vi "factorial function-for-while.vi"() -> ()   [LabVIEW 2023]
panel:
  out "String 2":string
  out "String":string
  out "String":string
  out "Numeric 6":i32
  in  "Numeric 5":i32
  in  "Numeric 3":i32
  out "Numeric 4":i32
  out "Numeric 2":i32
  in  "Numeric":i32
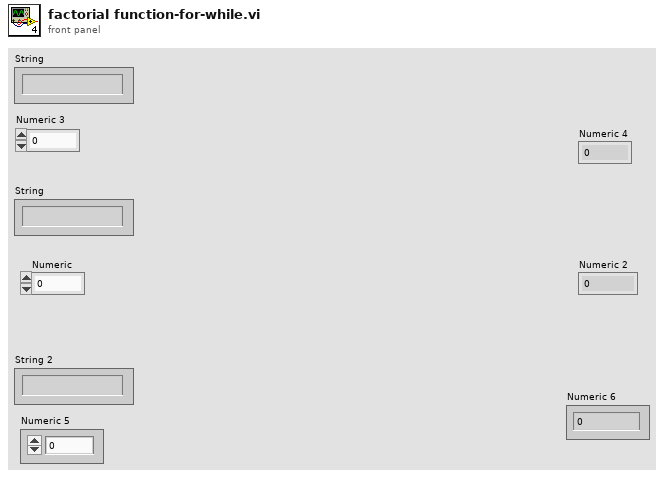
[diagram p1: front panel]
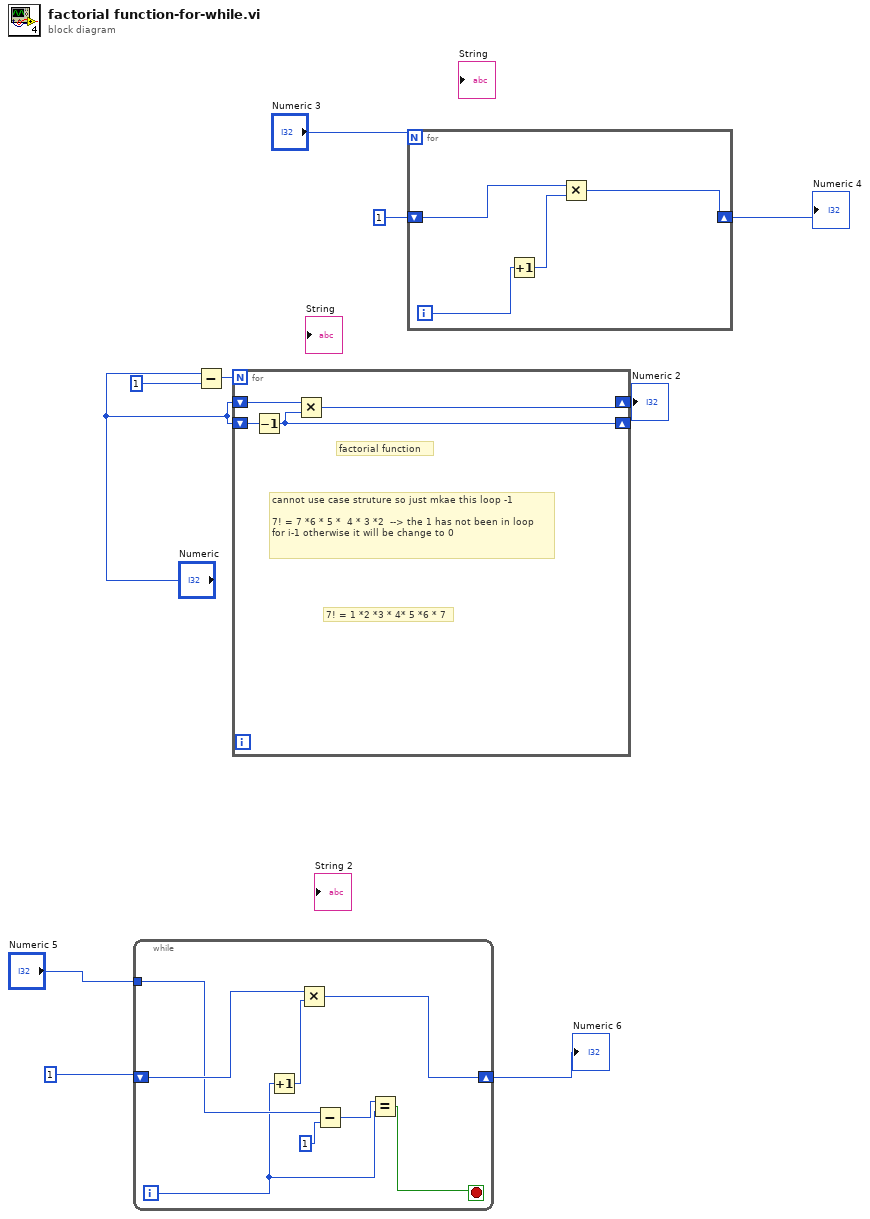
[diagram p0: block diagram]
diagram:
  # "factorial function"
  n1 = while {
    shift-right: [w16] -> w1
    shift-left: 1 -> [w17]
    tunnel: "Numeric 5" -> [w14]
    i -> [w11]
    stop <- w18 stop-if-true
    n2 = Increment(x=w11) -> (x+1=w15:i32)
    n3 = Multiply(x=w17, y=w15) -> (x*y=w16:i32)
    n4 = Subtract(x=w14, y=1) -> (x-y=w12:i32)
    n5 = Equal?(x=w12, y=w11) -> (x = y?=w18:bool)
  }
  "Numeric 6" <- w1
  n6 = Subtract(x="Numeric", y=1) -> (x-y=w8:i32)
  n7 = for {
    N: w8 -> [_]
    shift-right: [w21] -> w10
    shift-left: "Numeric" -> [w20]
    shift-right: [w19] -> _
    shift-left: "Numeric" -> [w22]
    # "7! = 1 *2 *3 * 4* 5 *6 * 7"
    # "cannot use case struture so just mkae this loop -1 \n\n7! = 7 *6 * 5 *  4 * 3 *2  --> the 1 has not been in loop\nfor i-1 otherwise it will be change to 0"
    n8 = Decrement(x=w22) -> (x-1=w19:i32)
    n9 = Multiply(x=w20, y=w19) -> (x*y=w21:i32)
  }
  "Numeric 2" <- w10
  n10 = for {
    N: "Numeric 3" -> [_]
    shift-right: [w23] -> w4
    shift-left: 1 -> [w25]
    i -> [w26]
    n11 = Increment(x=w26) -> (x+1=w24:i32)
    n12 = Multiply(x=w25, y=w24) -> (x*y=w23:i32)
  }
  "Numeric 4" <- w4
